vi "svfa_dBrefA to dBrefB.vi"(0 "input signal":dbl[](array[numeric]) format="%.2f", 1 "dB reference (desired)":dbl format="%.2f", 5 "linear/dB":enum16{"linear", "dB"}(ring), 7 "power/magnitude":enum16{"power", "magnitude"}(ring), 9 "view":enum16{"rms", "peak", "peak-peak"}(ring), 11 "dB reference":dbl format="%.2f") -> (4 "converted signal":dbl[](array[numeric]) format="%.2f", 6 "linear/dB (dupl)":enum16{"linear", "dB"}(ring), 8 "power/magnitude (dupl)":enum16{"power", "magnitude"}(ring), 10 "dup view":enum16{"rms", "peak", "peak-peak"}(ring), 15 "dB reference (out)":dbl format="%.2f")   [LabVIEW 2017]
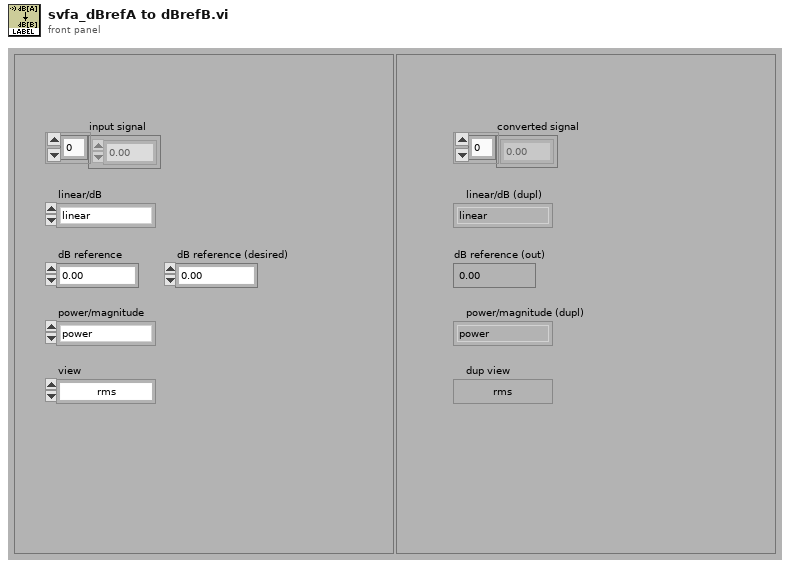
[diagram p1: front panel]
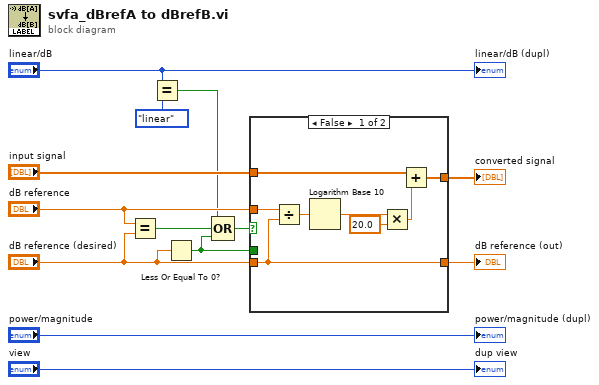
[diagram p0: block diagram]
diagram:
  n1 = Equal?(x="dB reference", y="dB reference (desired)") -> (x = y?=w5:bool)
  n2 = Equal?(x="linear/dB", y=enum16{"linear", "dB"}."linear" ("linear/dB")) -> (x = y?=w4:bool)
  n3 = Less Or Equal To 0?(x="dB reference (desired)") -> (x <= 0?=w1:bool)
  n4 = Compound Arithmetic op=OR(w4, w5, w1) -> (w3:bool)
  n5 = case shown="False" w3 {
    tunnel: "dB reference" -> [w21 w24]
    tunnel: "dB reference (desired)" -> [w17 w23]
    tunnel: "input signal" -> [w19 w26]
    tunnel: [w18 w26] -> w12
    tunnel: [w17 w22] -> w10
    tunnel: w1 -> [_ w25]
    frame False {
      n6 = Divide(x=w21, y=w17) -> (x/y=w20:dbl)
      n7 = Logarithm Base 10(1:w20) -> (0:w15:dbl)
      n8 = Multiply(x=w15, y=20.0 ("x")) -> (x*y=w16:dbl)
      n9 = Add(x=w19, y=w16) -> (x+y=w18:dbl[])
    }
    frame True {
      n10 = case shown="True" w25 {
        tunnel: w24 -> [_ w28]
        tunnel: w23 -> [w27 _]
        tunnel: [w27 w28] -> w22
        frame False {
        }
        frame True {
        }
      }
    }
  }
  "converted signal" <- w12
  "dB reference (out)" <- w10
  "linear/dB (dupl)" <- "linear/dB"
  "power/magnitude (dupl)" <- "power/magnitude"
  "dup view" <- "view"
